vi "clear_plot_selection.vi"(9 "# Lines Plot":i32, 11 "Plot Tree":refnum<vi>) -> ()   [LabVIEW 2019]
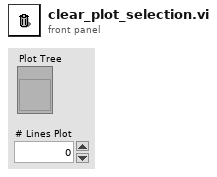
[diagram p1: front panel]
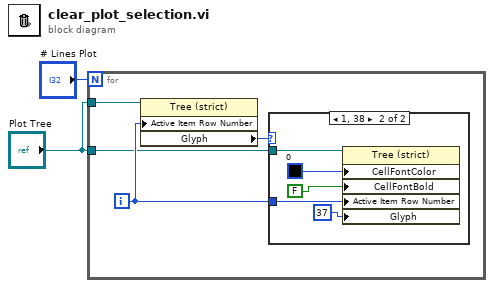
[diagram p0: block diagram]
diagram:
  n1 = for {
    N: "# Lines Plot" -> [_]
    tunnel: "Plot Tree" -> [w4]
    tunnel: "Plot Tree" -> [w3]
    i -> [w5]
    n2 = property on="Property Node" class="Tree (strict)"(reference=w3, "Active Item Row Number"=w5) -> ("Glyph"=w6:i32)  [unwired: 1 in, 2 out]
    n3 = case shown="1, 38" w6 {
      tunnel: w5 -> [_ w10]
      tunnel: w4 -> [_ w9]
      frame 15, 37, Default {
      }
      frame 1, 38 {
        n4 = property on="Property Node" class="Tree (strict)"(reference=w9, "CellFontColor"=u32 0 ("Active Cell:Cell Font:Color"), "CellFontBold"=FALSE ("Active Cell:Cell Font:Bold"), "Active Item Row Number"=w10, "Glyph"=37 ("Active Item:Symbol Index")) -> ()  [unwired: 1 in, 2 out]
      }
    }
  }
